vi "XYGrid.vi"() -> ()   [LabVIEW 2013]
panel:
  in  "Degrees":dbl
  out "XY Graph 2":cluster{"Y":dbl[], "Y":dbl[]}[](graph)=[{"Y"=[407.17179469133873], "Y"=[562.0]}]
  in  "y":dbl
  in  "x":dbl
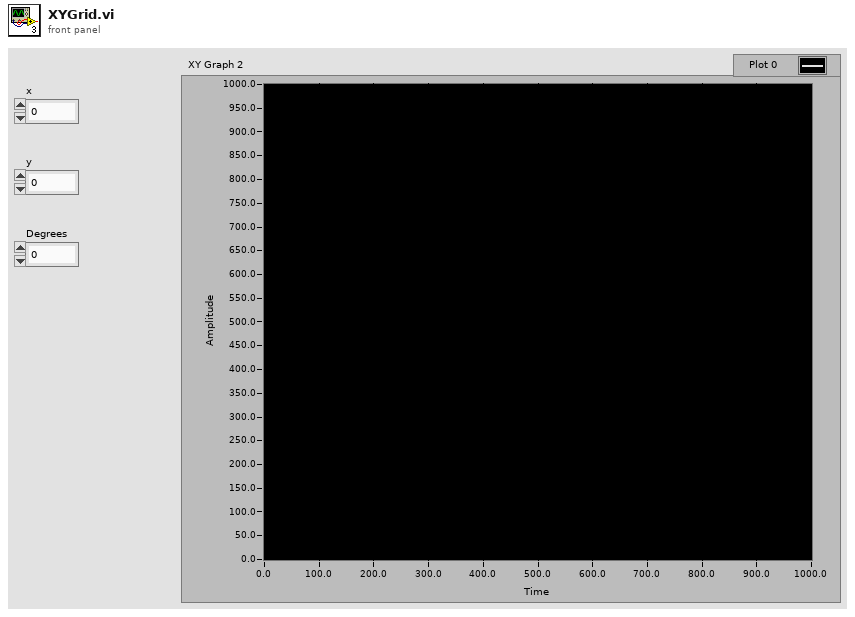
[diagram p1: front panel]
types:
  T1 = enum16{"0", "1", "2", "3", "4", "5", "6", "7", "8", "9", "A", "B", "C", "D", "E", "F", "G", "H", "I", "J", "K", "L", "M", "N", "O", "P", "Q", "R", "S", "T", "U", "V", "W", "X", "Y", "Z", "F1", "F2", "F3", "F4", "F5", "F6", "F7", "F8", "F9", "F10", "F11", "F12", "F13", "F14", "F15", "ADD", "BACK", "BACKSLASH", "CAPITAL", "COMMA", "DECIMAL", "DELETE", "DIVIDE", "DOWN", "END", "EQUALS", "ESCAPE", "GRAVE (`)", "HOME", "INSERT", "LBRACKET", "LCONTROL", "LEFT", "L ALT", "LSHIFT", "LWIN", "MINUS", "MULTIPLY", "NEXT", "NUMLOCK", "NUMPAD_0", "NUMPAD_1", "NUMPAD_2", "NUMPAD_3", "NUMPAD_4", "NUMPAD_5", "NUMPAD_6", "NUMPAD_7", "NUMPAD_8", "NUMPAD_9", "PAUSE", "PERIOD", "PRIOR (PG UP)", "RBRACKET", "RCONTROL", "RETURN", "RIGHT", "R ALT", "RSHIFT", "RWIN", "SCROLL", "SEMICOLON", "SLASH", "SPACE", "SUBTRACT", "TAB", "UP", "ENTER (num pad)", "' (quote)"}
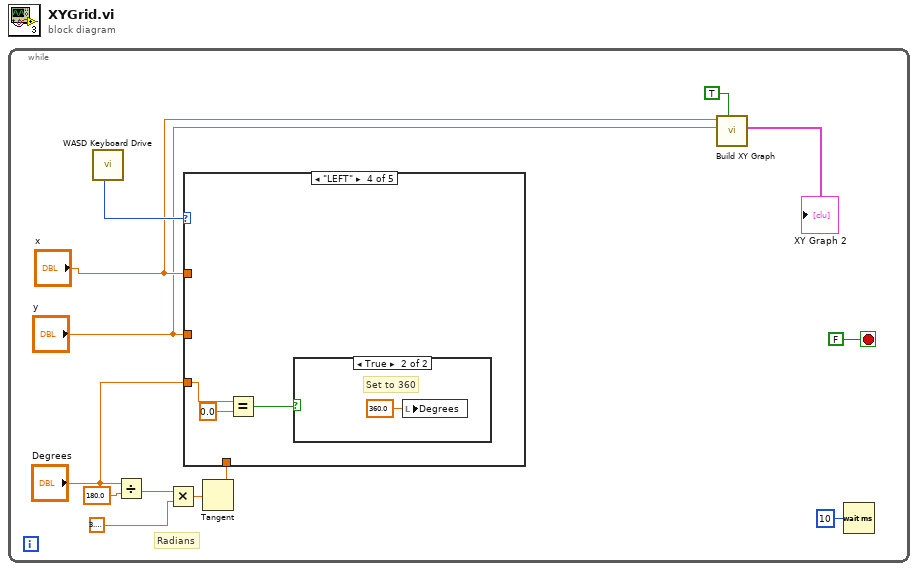
[diagram p0: block diagram]
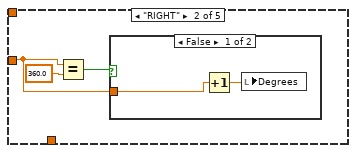
[diagram p3: hidden frame]
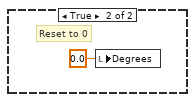
[diagram p4: hidden frame]
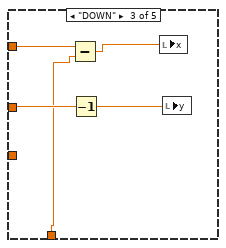
[diagram p5: hidden frame]
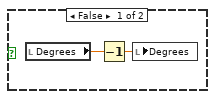
[diagram p6: hidden frame]
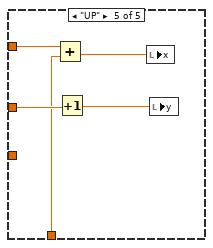
[diagram p7: hidden frame]
diagram:
  n1 = while {
    stop <- FALSE stop-if-true
    # "Radians"
    n2 = call "WASD Keyboard Drive.vi"() -> ("key"=w9:T1)  [unwired: 5 in, 2 out]
    n3 = Divide(x="Degrees", y=180.0) -> (x/y=w5:dbl)
    n4 = Multiply(x=w5, y=3.141592653589793) -> (x*y=w1:dbl)
    n5 = Tangent(1:w1) -> (0:w3:dbl)
    n6 = case shown="\"LEFT\"" w9 {
      tunnel: "x" -> [_ _ w22 _ w33]
      tunnel: "y" -> [_ _ w24 _ w35]
      tunnel: "Degrees" -> [_ w14 _ w27 _]
      tunnel: w3 -> [_ _ w21 _ w31]
      frame "0", Default {
      }
      frame "RIGHT" {
        n7 = Equal?(x=w14, y=360.0) -> (x = y?=w15:bool)
        n8 = case shown="False" w15 {
          tunnel: w14 -> [w17 _]
          frame False {
            n9 = Increment(x=w17) -> (x+1=w18:dbl)
            n10 = local write "Degrees"(w18) -> ()
          }
          frame True {
            # "Reset to 0"
            n11 = local write "Degrees"(0.0 ("Degrees")) -> ()
          }
        }
      }
      frame "DOWN" {
        n12 = Subtract(x=w22, y=w21) -> (x-y=w20:dbl)
        n13 = Decrement(x=w24) -> (x-1=w23:dbl)
        n14 = local write "x"(w20) -> ()
        n15 = local write "y"(w23) -> ()
      }
      frame "LEFT" {
        n16 = Equal?(x=w27, y=0.0) -> (x = y?=w25:bool)
        n17 = case shown="True" w25 {
          frame False {
            n18 = local read "Degrees"() -> (w29:dbl)
            n19 = Decrement(x=w29) -> (x-1=w28:dbl)
            n20 = local write "Degrees"(w28) -> ()
          }
          frame True {
            # "Set to 360"
            n21 = local write "Degrees"(360.0 ("Degrees")) -> ()
          }
        }
      }
      frame "UP" {
        n22 = Add(x=w33, y=w31) -> (x+y=w32:dbl)
        n23 = Increment(x=w35) -> (x+1=w34:dbl)
        n24 = local write "x"(w32) -> ()
        n25 = local write "y"(w34) -> ()
      }
    }
    n26 = call "Build XY Graph"("Enable"=TRUE, "Y Input"="y", "X Input"="x") -> ("XY Graph"=→"XY Graph 2":cluster{"X":dbl[], "Y":dbl[]}[])  [unwired: 7 in, 1 out]
    n27 = Wait (ms)(milliseconds to wait=u32 10) -> ()  [unwired: 1 out]
  }
